vi "ukol3.vi"() -> ()   [LabVIEW 2023]
uses:
  <vilib>/Analysis/2dsp.llb/1D Convolution (DBL).vi
  <vilib>/Utility/file.llb/Read Delimited Spreadsheet (DBL).vi
  <vilib>/Analysis/NI_AALBase.lvlib
  <vilib>/Analysis/NI_AALPro.lvlib
panel:
  out "Waveform Graph 3":dbl[](graph)
  out "Waveform Graph 2":dbl[](graph)
  out "Waveform Graph":dbl[](graph)
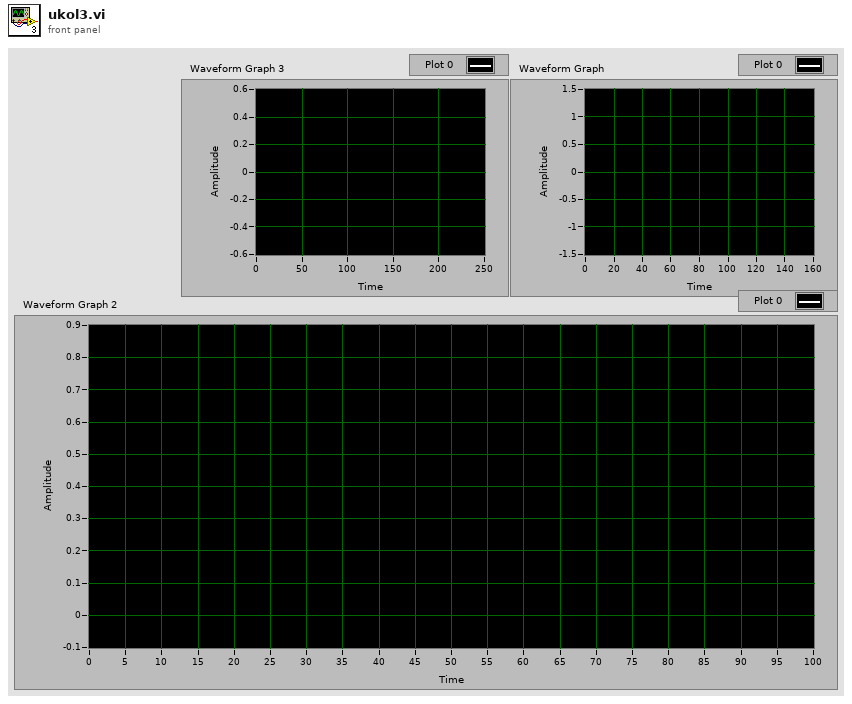
[diagram p1: front panel]
types:
  T1 = cluster{"frequency":dbl, "amplitude":dbl, "phase":dbl}[]
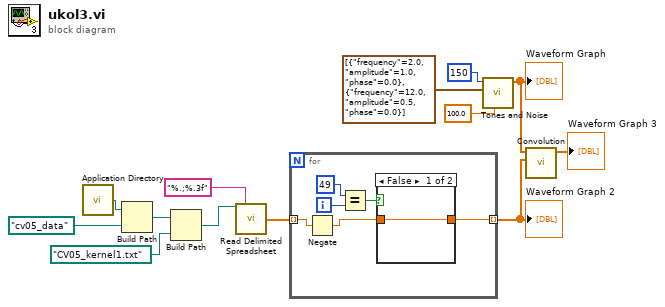
[diagram p0: block diagram]
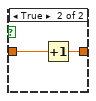
[diagram p2: hidden frame]
diagram:
  n1 = call <vilib>:"Application Directory.vi"() -> ("Application Directory"=w10:path)
  n2 = Build Path(base path=w10, name or relative path=path "cv05_data") -> (appended path=w8:path)
  n3 = Build Path(base path=w8, name or relative path=path "CV05_kernel1.txt") -> (appended path=w6:path)
  n4 = call-poly <vilib>:"Read Delimited Spreadsheet.vi"("file path (dialog if empty)"=w6, "format (%.3f)"="%.;%.3f") -> ("first row"=w4:dbl[])  [unwired: 8 in, 5 out]
  n5 = for {
    tunnel: w4 -> [w14] mode=indexing
    tunnel: [w16] -> w1 mode=indexing
    i -> [w19]
    n6 = Negate(x=w14) -> (-x=w15:dbl)
    n7 = Equal?(x=49, y=w19) -> (x = y?=w17:bool)
    n8 = case shown="False" w17 {
      tunnel: [w20 w22] -> w16
      tunnel: w15 -> [w20 w21]
      frame False {
      }
      frame True {
        n9 = Increment(x=w21) -> (x+1=w22:dbl)
      }
    }
  }
  "Waveform Graph 2" <- w1
  n10 = call <vilib>:"Tones and Noise.vi"("Fs"=100.0, "tones"=T1 [{"frequency"=2.0, "amplitude"=1.0, "phase"=0.0}, {"frequency"=12.0, "amplitude"=0.5, "phase"=0.0}], "samples"=150) -> ("tones and noise"=w3:dbl[])  [unwired: 7 in, 1 out]
  "Waveform Graph" <- w3
  n11 = call-poly <vilib>:"Convolution.vi"("Y"=w1, "X"=w3) -> ("X * Y"=→"Waveform Graph 3":dbl[])  [unwired: 8 in, 1 out]
